vi "MouseMove Response.vi"(7 "Dragging":bool, 8 "error in (no error)":errorcluster, 9 "Current Coords":T1, 10 "Delta":T1, 11 "Editor Handler in":refnum<class "Image Editor Handler.lvclass">) -> (0 "error out":errorcluster, 2 "Refresh?":bool, 3 "Editor Handler out":refnum<class "Image Editor Handler.lvclass">)   [LabVIEW 2017, in "LV Image Editor Framework.lvlib" / "Image Editor Handler.lvclass"]
uses:
  Image Editor Handler.lvclass
  <vilib>/Utility/miscctls.llb/LVPoint32TypeDef.ctl
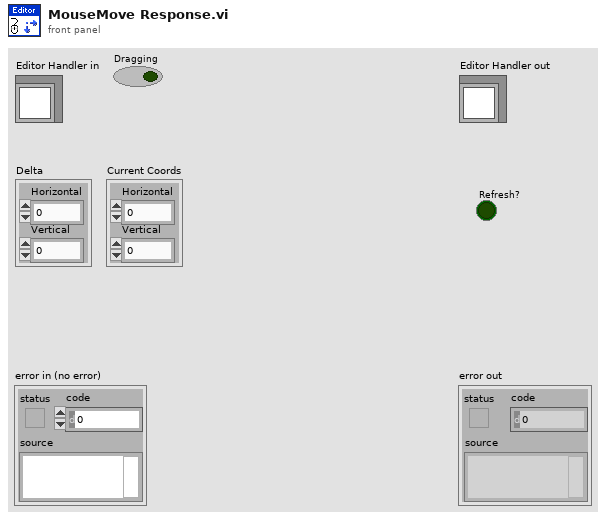
[diagram p1: front panel]
types:
  T1 = typedef "LVPoint32TypeDef.ctl" = cluster{"Horizontal":i32, "Vertical":i32}
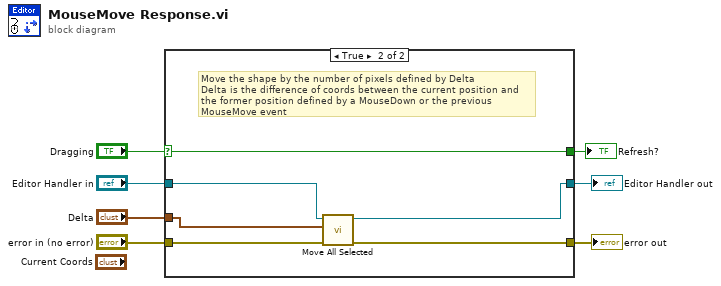
[diagram p0: block diagram]
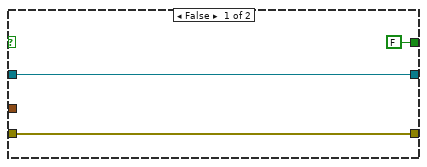
[diagram p2: hidden frame]
diagram:
  n1 = case shown="True" "Dragging" {
    selector: "Dragging" -> [_ w11]
    tunnel: [w10 w12] -> w6
    tunnel: [w9 w15] -> w5
    tunnel: "Editor Handler in" -> [w9 w16]
    tunnel: "Delta" -> [_ w14]
    tunnel: "error in (no error)" -> [w10 w13]
    tunnel: [FALSE w11] -> w1
    frame False {
    }
    frame True {
      # "Move the shape by the number of pixels defined by Delta\nDelta is the difference of coords between the current position and the former position defined by a MouseDown or the previous MouseMove event"
      n2 = call "Move All Selected.vi"("error in (no error)"=w13, "Delta"=w14, "Editor Handler in"=w16) -> ("error out"=w12:errorcluster, "Editor Handler out"=w15:refnum<class "Image Editor Handler.lvclass">)  [unwired: 7 in]
    }
  }
  "error out" <- w6
  "Editor Handler out" <- w5
  "Refresh?" <- w1
